vi "Measure Voltage.vi"(7 "Chanel":string, 11 "VISA Source":string) -> (3 "Response":dbl, 4 "error out":errorcluster)   [LabVIEW 2020]
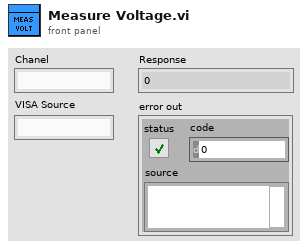
[diagram p1: front panel]
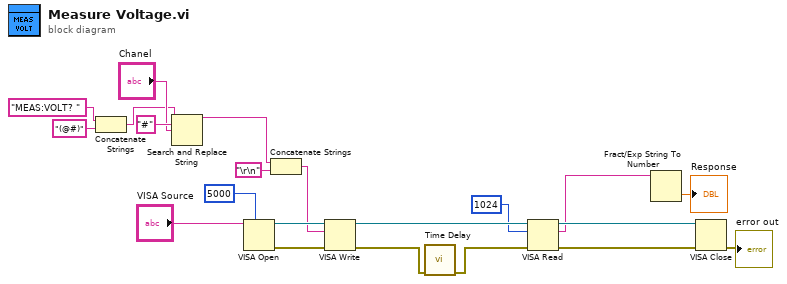
[diagram p0: block diagram]
diagram:
  n1 = Concatenate Strings("MEAS:VOLT? " ("string"), "(@#)" ("string")) -> (w9:string)
  n2 = Search and Replace String(input string=w9, search string="#", replace string="Chanel") -> (result string=w8:string)  [unwired: 5 in, 3 out]
  n3 = VISA Open(timeout (0)=u32 5000 ("VISA Open timeout (0)"), VISA resource name="VISA Source") -> (VISA resource name=w21:refnum<visa-resource-name>, error out=w20:errorcluster)  [unwired: 3 in]
  n4 = Concatenate Strings(w8, "\r\n") -> (w14:string)
  n5 = VISA Write(VISA resource name=w21, write buffer=w14, error in (no error)=w20) -> (VISA resource name out=w16:refnum<visa-resource-name>, error out=w5:errorcluster)  [unwired: 1 out]
  n6 = call "Time Delay"("error in (no error)"=w5) -> ("error out"=w4:errorcluster)  [unwired: 10 in]
  n7 = VISA Read(VISA resource name=w16, byte count=u32 1024, error in (no error)=w4) -> (VISA resource name out=w19:refnum<visa-resource-name>, read buffer=w3:string, error out=w18:errorcluster)  [unwired: 1 out]
  n8 = Fract/Exp String To Number(string=w3) -> (number=→"Response":dbl)  [unwired: 3 in, 1 out]
  n9 = VISA Close(VISA resource name=w19, error in (no error)=w18) -> (error out=→"error out":errorcluster)
